vi "Initialize.vi"(6 "Default return":variant, 7 "writer buffer size":i32=4096, 8 "error in (no error)":errorcluster, 9 "writer url":string, 10 "reader name":string) -> (0 "error out":errorcluster, 3 "NetworkStreamWriter out":refnum<class "NetworkStreamReader.lvclass">)   [LabVIEW 2011, in "NetworkStreamReader.lvclass"]
doc: "This VI returns an instance of the NetworkStreamReader class. A NetworkStreamReader attempts to open a network stream with a writer endpoint. As with network streams, the writer url on the reader or the reader url on the writer must be given before the connection can be made. Note that until a connection is made, this VI will not return. It will, however, stop on a commanded e-stop from the top-level VI. This VI also launches a reader daemon which constantly adds information passed across the stream to an internal queue accessed by the Read method."
uses:
  NetworkStreamReader.lvclass
  Shared/message.ctl
  Shared/messageQueue.ctl
  NetworkStreamReader.lvclass/NetworkStreamReader.ctl
  ReaderDaemon.vi
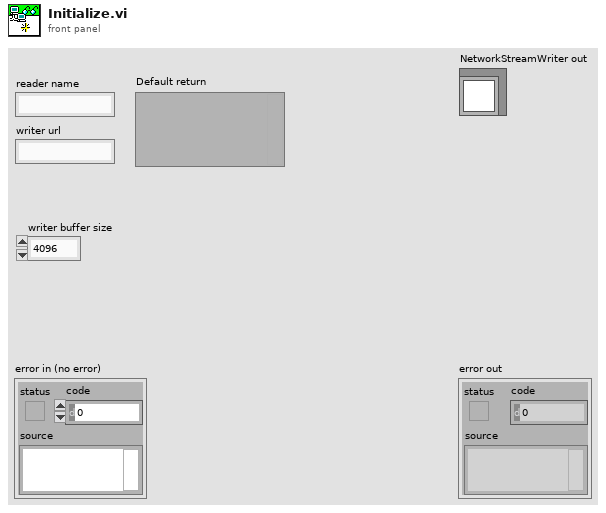
[diagram p1: front panel]
types:
  T1 = typedef "message.ctl" = cluster{"Data":variant, "Time since start (s)":dbl}
  T2 = typedef "messageQueue.ctl" = refnum<queue>
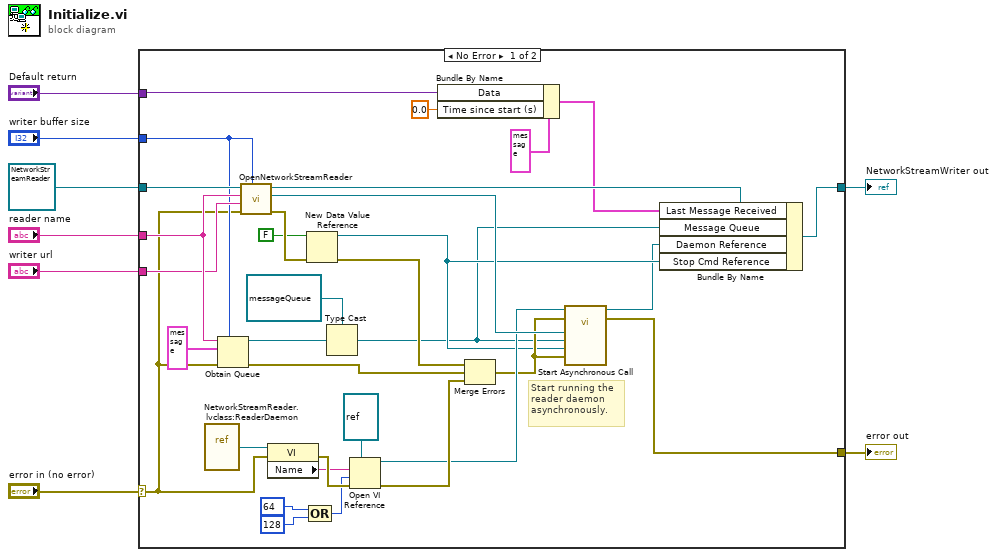
[diagram p0: block diagram]
diagram:
  n1 = case shown="No Error" "error in (no error)" {
    selector: "error in (no error)" -> [w30 w43]
    tunnel: [w26 w43] -> w7
    tunnel: [w36 w42] -> w6
    tunnel: refnum<class "NetworkStreamReader.lvclass"> refnum ("NetworkStreamWriter in") -> [w41 w42]
    tunnel: "reader name" -> [w40 _]
    tunnel: "writer url" -> [w39 _]
    tunnel: "writer buffer size" -> [w37 _]
    tunnel: "Default return" -> [w10 _]
    frame No Error {
      # "Start running the \nreader daemon\nasynchronously."
      n2 = vi-ref "NetworkStreamReader.lvclass:ReaderDaemon.vi"() -> (w31:refnum<vi>)
      n3 = Obtain Queue(max queue size (-1, unlimited)=w37, name (unnamed)=w40, element data type=T1 {"Data"=variant, "Time since start (s)"=0.0}, error in (no error)=w30) -> (queue out=w16:refnum<queue>, error out=w35:errorcluster)  [unwired: 1 in, 1 out]
      n4 = call "OpenNetworkStreamReader.vi"("reader buffer size"=w37, "error in (no error)"=w30, "writer url"=w39, "reader name"=w40, "NetworkStreamReader in"=w41) -> ("error out"=w21:errorcluster, "Reader Endpoint"=w28:refnum<k21>, "NetworkStreamReader out"=w13:refnum<class "NetworkStreamReader.lvclass">)  [unwired: 4 in]
      n5 = property class="VI"(reference=w31, error in=w30) -> (error out=w34:errorcluster, "Name"=w32:string)  [unwired: 1 out]
      n6 = New Data Value Reference(data value=FALSE, error in=w21) -> (data value reference=w18:refnum<data-value>, error out=w20:errorcluster)
      n7 = Compound Arithmetic op=OR(64 ("options"), 128 ("options")) -> (w23:i32)
      n8 = Type Cast(type=T2 refnum ("Variant Queue"), x=w16) -> (*(type *) &x=w14:T2)
      n9 = Open VI Reference(type specifier VI Refnum (for type only)=refnum<vi> refnum, vi path=w32, options=w23, error in (no error)=w34) -> (vi reference=w27:refnum<vi>, error out=w29:errorcluster)  [unwired: 2 in]
      n10 = Bundle By Name(cluster=T1 {"Data"=variant, "Time since start (s)"=0.0} ("Last Message Received"), "Data"=w10, "Time since start (s)"=0.0) -> (w9:T1)
      n11 = Merge Errors(w20, w35, w29) -> (w22:errorcluster)
      n12 = call-by-ref "Start Asynchronous Call"(reference=w27, error in=w22, 8:"error in (no error)"=w22, "Stop command reference"=w18, "Variant Queue"=w14, "Reader Endpoint"=w28) -> (reference out=w17:refnum<vi>, error out=w26:errorcluster)  [unwired: 8 in]
      n13 = Bundle By Name(cluster=w13, "Last Message Received"=w9, "Message Queue"=w14, "Daemon Reference"=w17, "Stop Cmd Reference"=w18) -> (w36:refnum<class "NetworkStreamReader.lvclass">)
    }
    frame Error {
    }
  }
  "error out" <- w7
  "NetworkStreamWriter out" <- w6
